vi "tcp_read_length.vi"(8 "error in (no error)":errorcluster, 9 "timeout ms (10000)":i32=10000, 11 "conn in":refnum<k5>) -> (0 "error out":errorcluster, 1 "response":string, 2 "token":u64 format="%016x", 3 "conn out":refnum<k5>)   [LabVIEW 2017, in "rethinkdb.lvlib"]
uses:
  rethinkdb.lvlib
  debug_action.ctl
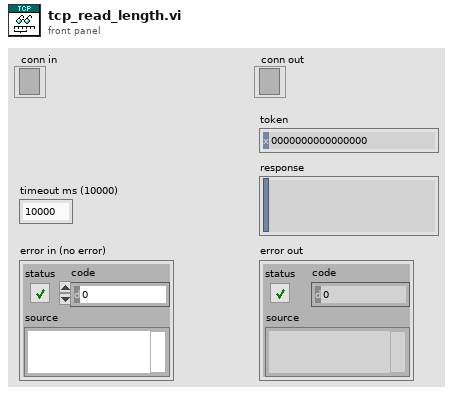
[diagram p1: front panel]
types:
  T1 = typedef "rethinkdb.lvlib/debug_action.ctl" = enum8{"get", "set_query", "set_response", "clear"}
  T2 = enum16{"Standard", "Buffered", "CRLF", "Immediate"}
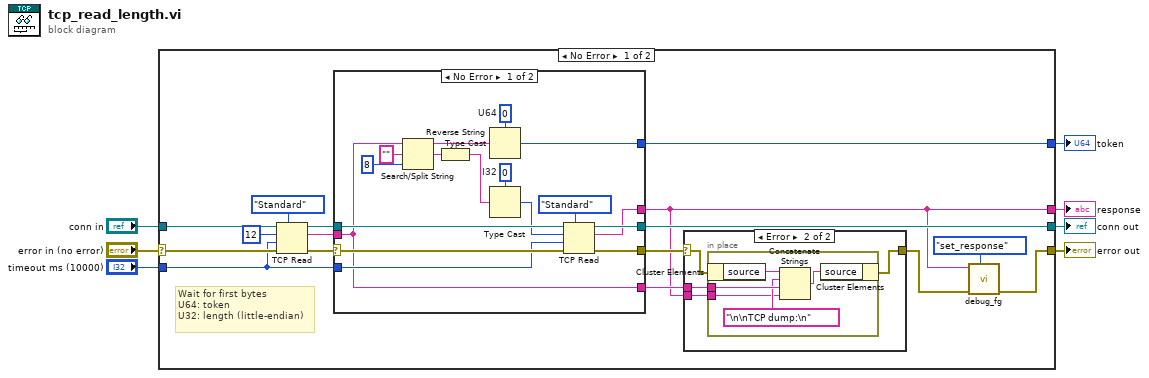
[diagram p0: block diagram]
diagram:
  n1 = case shown="No Error" "error in (no error)" {
    selector: "error in (no error)" -> [w22 w55]
    tunnel: "conn in" -> [w23 w54]
    tunnel: "timeout ms (10000)" -> [w14 _]
    tunnel: [w10 w55] -> w4
    tunnel: [w18 w54] -> w3
    tunnel: [w8 _] -> w2
    tunnel: [w12 _] -> w1
    frame No Error {
      # "Wait for first bytes\nU64: token\nU32: length (little-endian)"
      n2 = TCP Read(connection ID=w23, bytes to read=12, error in (no error)=w22, 7:T2."Standard" ("mode (standard)"), 9:w14) -> (connection ID out=w17:refnum<k5>, data out=w16:string, error out=w19:errorcluster)
      n3 = case shown="No Error" w19 {
        selector: w19 -> [w40 w43]
        tunnel: [w26 w43] -> w15
        tunnel: [w38 w42] -> w18
        tunnel: w17 -> [w39 w42]
        tunnel: w16 -> [w25 w41]
        tunnel: [w27 _] -> w8
        tunnel: w14 -> [w37 _]
        tunnel: [w25 w41] -> w13
        tunnel: [w24 _] -> w12
        frame No Error {
          w32 = 0  # I32
          w33 = u64 0  # U64
          n4 = Search/Split String(string=w25, search string/char (-)="", offset (0)=8) -> (substring before match=w34:string, match + rest of string=w31:string)  [unwired: 1 out]
          n5 = Reverse String(1:w31) -> (0:w30:string)
          n6 = Type Cast(type=w33, x=w34) -> (*(type *) &x=w24:u64)
          n7 = Type Cast(type=w32, x=w30) -> (*(type *) &x=w28:i32)
          n8 = TCP Read(connection ID=w39, bytes to read=w28, error in (no error)=w40, 7:T2."Standard" ("mode (standard)"), 9:w37) -> (connection ID out=w38:refnum<k5>, data out=w27:string, error out=w26:errorcluster)
        }
        frame Error {
        }
      }
      n9 = case shown="Error" w15 {
        selector: w15 -> [w44 w46]
        tunnel: w13 -> [_ w48]
        tunnel: [w44 w47] -> w9
        tunnel: w8 -> [_ w45]
        frame No Error {
        }
        frame Error {
          n10 = in-place {
            in-place-border: w48 -> [w51]
            in-place-border: w45 -> [w49]
            n11 = in-place-cluster #1(w46) -> ("source"=w53:string)
            n12 = Concatenate Strings(w53, "\n\nTCP dump:\n" ("format string"), w51, w49) -> (w52:string)
            n13 = in-place-cluster #1("source"=w52) -> (w47:errorcluster)
          }
        }
      }
      n14 = call "debug_fg.vi"("action"=debug_action."set_response", "error in (no error)"=w9, "data"=w8) -> ("error out"=w10:errorcluster)  [unwired: 7 in, 1 out]
    }
    frame Error {
    }
  }
  "error out" <- w4
  "conn out" <- w3
  "response" <- w2
  "token" <- w1
